vi "Send.vi"(7 "Priority":enum16{""}(ring) caption="Message Priority (Normal)", 8 "error in (no error)":errorcluster, 11 "Message Enqueuer in":refnum<class>) -> (0 "error out":errorcluster, 3 "Message Enqueuer out":refnum<class>)   [LabVIEW 2023, in "Message Template Interface.lvclass"]
uses:
  Message Template Interface.lvclass
  Message Template Interface.lvclass/Message Template Interface.ctl
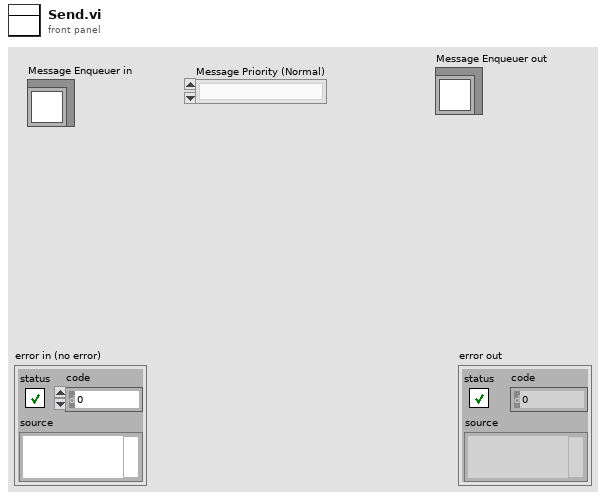
[diagram p1: front panel]
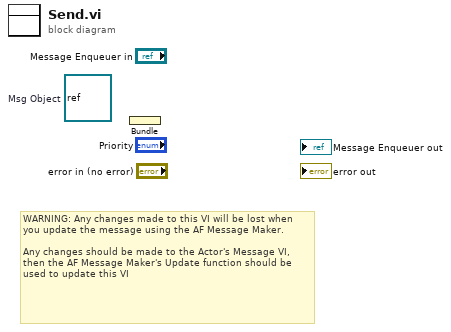
[diagram p0: block diagram]
diagram:
  (unwired) refnum<class> refnum  # Msg Object
  # "WARNING: Any changes made to this VI will be lost when you update the message using the AF Message Maker.\n\nAny changes should be made to the Actor's Message VI, then the AF Message Maker's Update function should be used to update this VI"
  n1 = Bundle "Bundle"() -> ()  [unwired: 2 in, 1 out]
